vi "WriteElog.vi"(5 "Elog Type (eg MicrowaveLog)":string, 7 "Elog Encodeing":T1=enum."PLAIN", 8 "error in (no error)":errorcluster, 9 "Elog Message":string, 11 "Attributes (ie \nAuthor=Fred Dibna, \nSubject=Really important announcement)":string[](array[string])) -> (0 "Error Out":errorcluster)   [LabVIEW 2018, in "feGEM DataPacker.lvlib"]
uses:
  feGEM DataPacker.lvlib
  DataPacker/Utilities/ElogEncoding.ctl
  b6a75a92-8101-4402-9ca7-c715011fb302.vi
  b6a75a92-8101-4402-9ca7-c715011fb302.vi/55764636-801d-4e38-9be8-6b44cc230144.vi
panel:
  out "Combined String for MIDAS":string
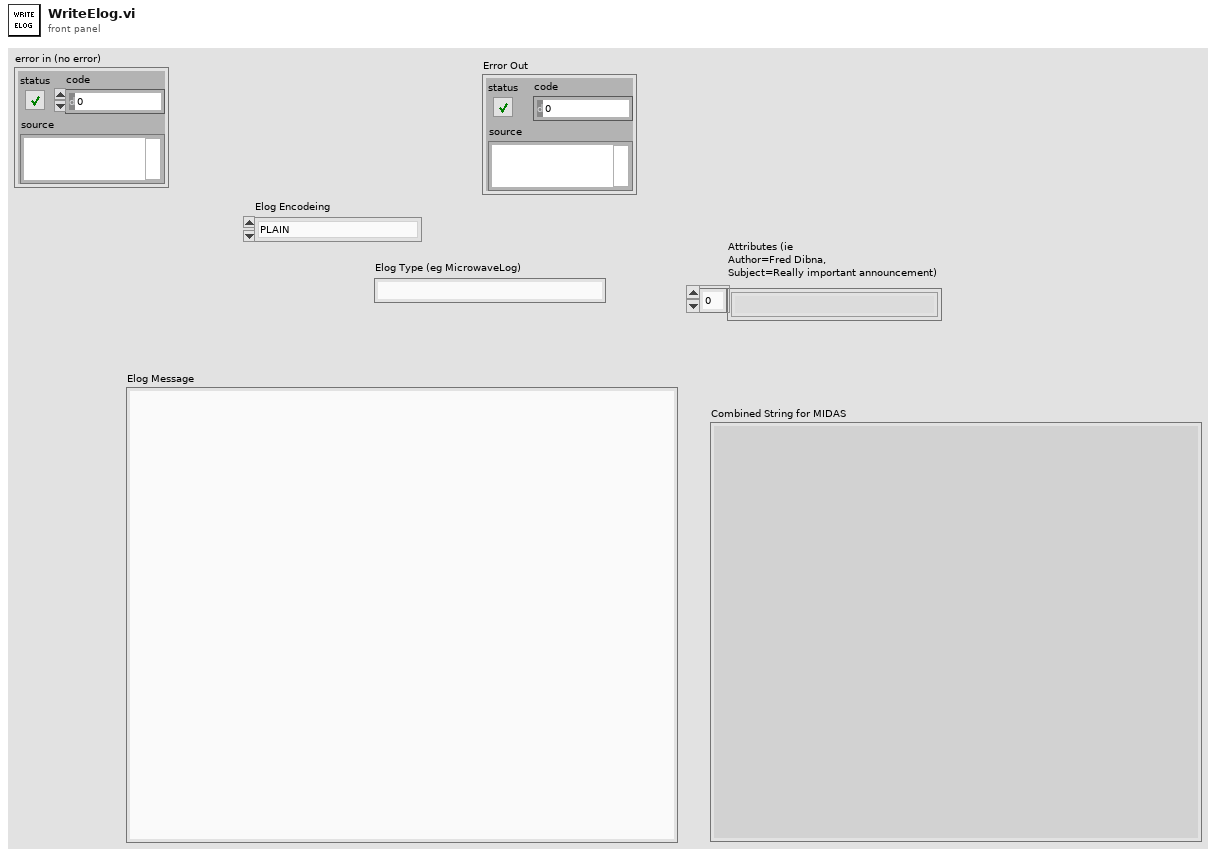
[diagram p1: front panel]
types:
  T1 = typedef "feGEM DataPacker.lvlib/ElogEncoding.ctl" = enum16{"ELCODE", "PLAIN", "HTML"}
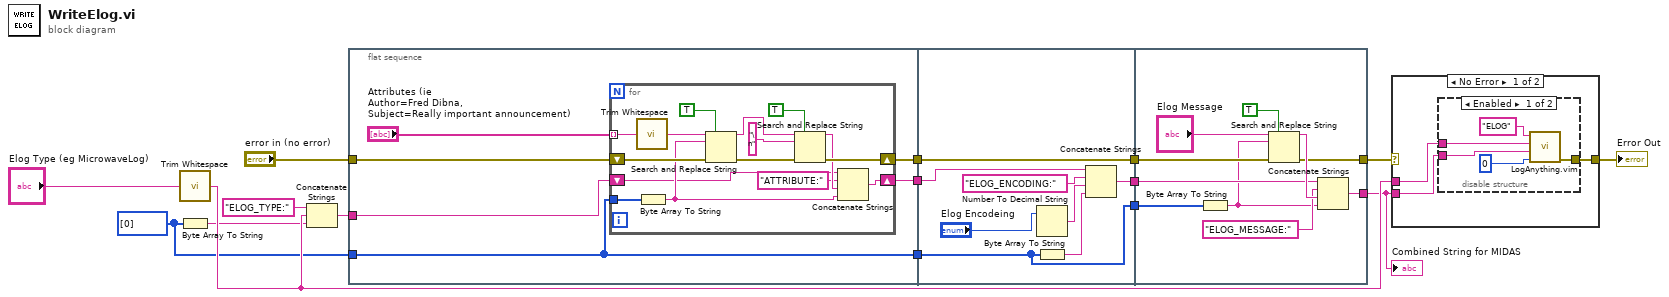
[diagram p0: block diagram]
diagram:
  w5 = u8[] [0] ("unsigned byte array")
  n1 = call <vilib>:"Trim Whitespace.vi"("string"="Elog Type (eg MicrowaveLog)") -> ("trimmed string"=w8:string)  [unwired: 1 in]
  n2 = Byte Array To String(unsigned byte array=w5) -> (string=w4:string)
  n3 = Concatenate Strings("ELOG_TYPE:" ("string"), w8, w4) -> (w14:string)
  n4 = flat-sequence {
    tunnel: w14 -> [w22]
    tunnel: w5 -> [w17]
    tunnel: "error in (no error)" -> [w21]
    tunnel: [w19] -> w3
    tunnel: [w18] -> w2
    tunnel: [w17] -> w1
    tunnel: [w38] -> w13
    tunnel: [w45] -> w12
    tunnel: [w39] -> w10
    tunnel: w3 -> [w40]
    tunnel: w2 -> [w39]
    tunnel: w1 -> [w38]
    tunnel: w13 -> [w47]
    tunnel: [w50] -> w7
    tunnel: w12 -> [w51]
    tunnel: w10 -> [w49]
    tunnel: [w48] -> w9
    frame #0 {
      n5 = for {
        tunnel: w17 -> [w30]
        tunnel: "Attributes (ie \nAuthor=Fred Dibna, \nSubject=Really important announcement)" -> [w29] mode=indexing
        shift-right: [w27] -> w18
        shift-left: w21 -> [w31]
        shift-right: [w28] -> w19
        shift-left: w22 -> [w24]
        n6 = call <vilib>:"Trim Whitespace.vi"("string"=w29) -> ("trimmed string"=w32:string)  [unwired: 1 in]
        n7 = Byte Array To String(unsigned byte array=w30) -> (string=w25:string)
        n8 = Search and Replace String(replace all?=TRUE ("replace all? (F)"), input string=w32, search string=w25, error in=w31) -> (result string=w36:string, error out=w37:errorcluster)  [unwired: 4 in, 2 out]
        n9 = Search and Replace String(replace all?=TRUE ("replace all? (F)"), input string=w36, search string="\n", error in=w37) -> (result string=w26:string, error out=w27:errorcluster)  [unwired: 4 in, 2 out]
        n10 = Concatenate Strings(w24, "ATTRIBUTE:" ("string"), w26, w25) -> (w28:string)
      }
    }
    frame #1 {
      n11 = Number To Decimal String(number="Elog Encodeing") -> (decimal integer string=w44:string)  [unwired: 1 in]
      n12 = Byte Array To String(unsigned byte array=w38) -> (string=w41:string)
      n13 = Concatenate Strings(w40, "ELOG_ENCODING:" ("string"), w44, w41) -> (w45:string)
    }
    frame #2 {
      n14 = Byte Array To String(unsigned byte array=w47) -> (string=w46:string)
      n15 = Search and Replace String(replace all?=TRUE ("replace all? (F)"), input string="Elog Message", search string=w46, error in=w49) -> (result string=w55:string, error out=w48:errorcluster)  [unwired: 4 in, 2 out]
      n16 = Concatenate Strings(w51, "ELOG_MESSAGE:" ("string"), w55, w46) -> (w50:string)
    }
  }
  n17 = case shown="No Error" w9 {
    selector: w9 -> [_ w64]
    tunnel: w8 -> [w58 _]
    tunnel: w7 -> [w57 _]
    tunnel: [w56 w64] -> w6
    frame No Error {
      n18 = disable-structure shown="Enabled" {
        disable-tunnel: w58 -> [w61 _]
        disable-tunnel: w57 -> [w60 _]
        disable-tunnel: [w59 _] -> w56
        frame Enabled {
          n19 = call "LogAnything.vim"("Period to update history plots (seconds)\nUnset (65535) = Use MIDAS default in ODB\n0 = Record but do not put in histories"=0 ("Rate to update history plots"), "Array"=w60, "Variable Name"=w61, "Category"="ELOG") -> ("error out"=w59:errorcluster)  [unwired: 6 in, 1 out]
        }
        frame Disabled {
        }
      }
    }
    frame Error {
    }
  }
  "Error Out" <- w6
  "Combined String for MIDAS" <- w7
